vi "Add Header ZIP Query.vi"(8 "error in":errorcluster, 10 "Api Token":string="8y3UfvlU-s_u9u_oxA6shSxOW3EspqNUnOF1NvG3HuRk3uhql6GwvIuXxEX0eFPkzaJQUr8iPPkS1eW6XzXgRw==", 11 "client handle in":T1) -> (0 "error out":errorcluster, 3 "client handle out":T1)   [LabVIEW 2020, in "InfluxDB v2 Client.lvlib"]
doc: "Creates the header for query"
uses:
  InfluxDB v2 Client.lvlib
  <vilib>/httpClient/ClientHandle.ctl
  <vilib>/httpClient/LabVIEWHTTPClient.lvlib
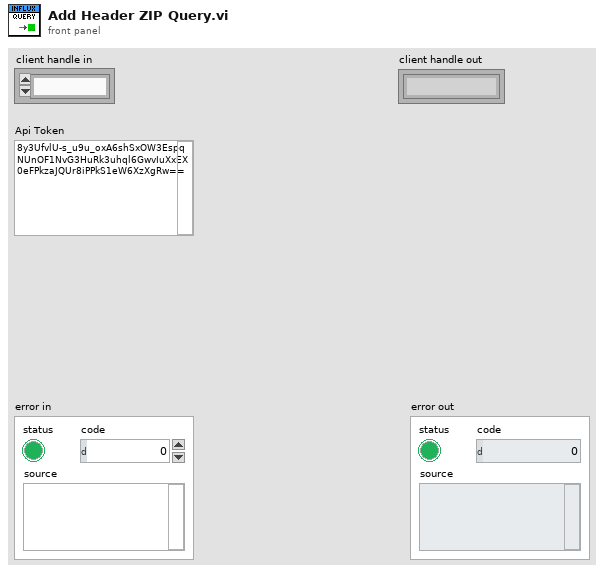
[diagram p1: front panel]
types:
  T1 = typedef "LabVIEWHTTPClient.lvlib/ClientHandle.ctl" = refnum<k1>
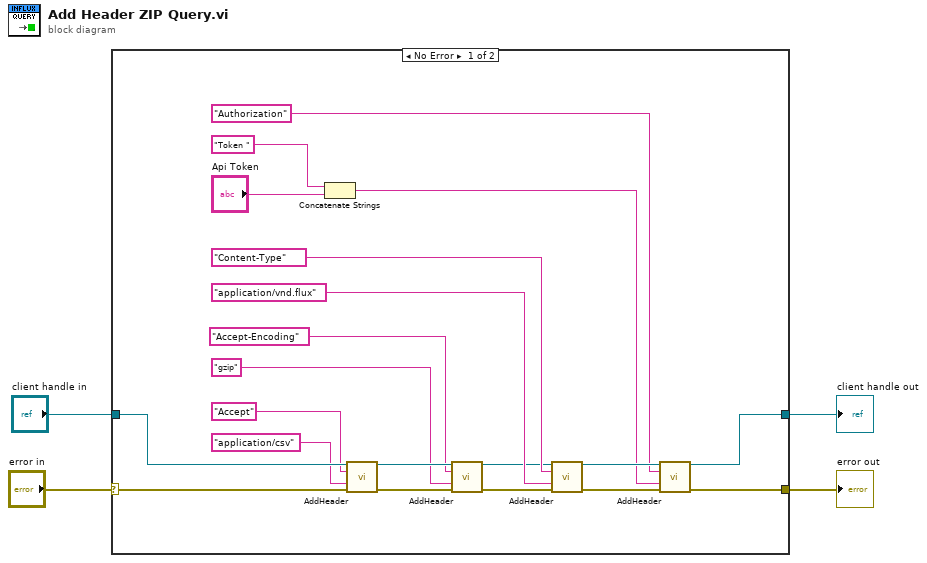
[diagram p0: block diagram]
diagram:
  n1 = case shown="No Error" "error in" {
    selector: "error in" -> [w14 w25]
    tunnel: [w17 w25] -> w3
    tunnel: "client handle in" -> [w13 w26]
    tunnel: [w15 w26] -> w1
    frame No Error {
      n2 = Concatenate Strings("Token ", "Api Token") -> (w18:string)
      n3 = call <vilib>:"AddHeader.vi"("client handle"=w13, "header"="Accept" ("value"), "value"="application/csv", "error in (no error)"=w14) -> ("client handle out"=w9:T1, "error out"=w10:errorcluster)  [unwired: 10 in]
      n4 = call <vilib>:"AddHeader.vi"("client handle"=w9, "header"="Accept-Encoding" ("value"), "value"="gzip", "error in (no error)"=w10) -> ("client handle out"=w8:T1, "error out"=w7:errorcluster)  [unwired: 10 in]
      n5 = call <vilib>:"AddHeader.vi"("client handle"=w8, "header"="Content-Type", "value"="application/vnd.flux", "error in (no error)"=w7) -> ("client handle out"=w22:T1, "error out"=w21:errorcluster)  [unwired: 10 in]
      n6 = call <vilib>:"AddHeader.vi"("client handle"=w22, "header"="Authorization", "value"=w18, "error in (no error)"=w21) -> ("client handle out"=w15:T1, "error out"=w17:errorcluster)  [unwired: 10 in]
    }
    frame Error {
    }
  }
  "client handle out" <- w1
  "error out" <- w3
